vi "niVNA_SParamMeasure_Demo.vi"() -> ()   [LabVIEW 2013]
uses:
  <vilib>/Analysis/baseanly.llb/Mean (DBL).vi
  <instrlib>/niVNA/niVNA.llb/niVNA Load Calibration And Configuration Data From File.vi
  <instrlib>/niVNA/niVNA.llb/niVNA Fetch Sweep Measurement Complex (CDB).vi
  <vilib>/Analysis/baseanly.llb/Mean (CDB).vi
  <vilib>/Analysis/NI_AALBase.lvlib
panel:
  in  "Stop Button":bool
  out "P2":dbl[](graph)
  out "P1":dbl[](graph)
  out "CPD":dbl[](graph)
  out "error out":errorcluster
  in  "SavedCalPath":path=path "C:/Users/Eddie.Rickey/Documents/RCV_PXI/Calibration/#Cal - VNA_ 50MHz.chx"
  in  "resource name":refnum<k15>="5632_0"
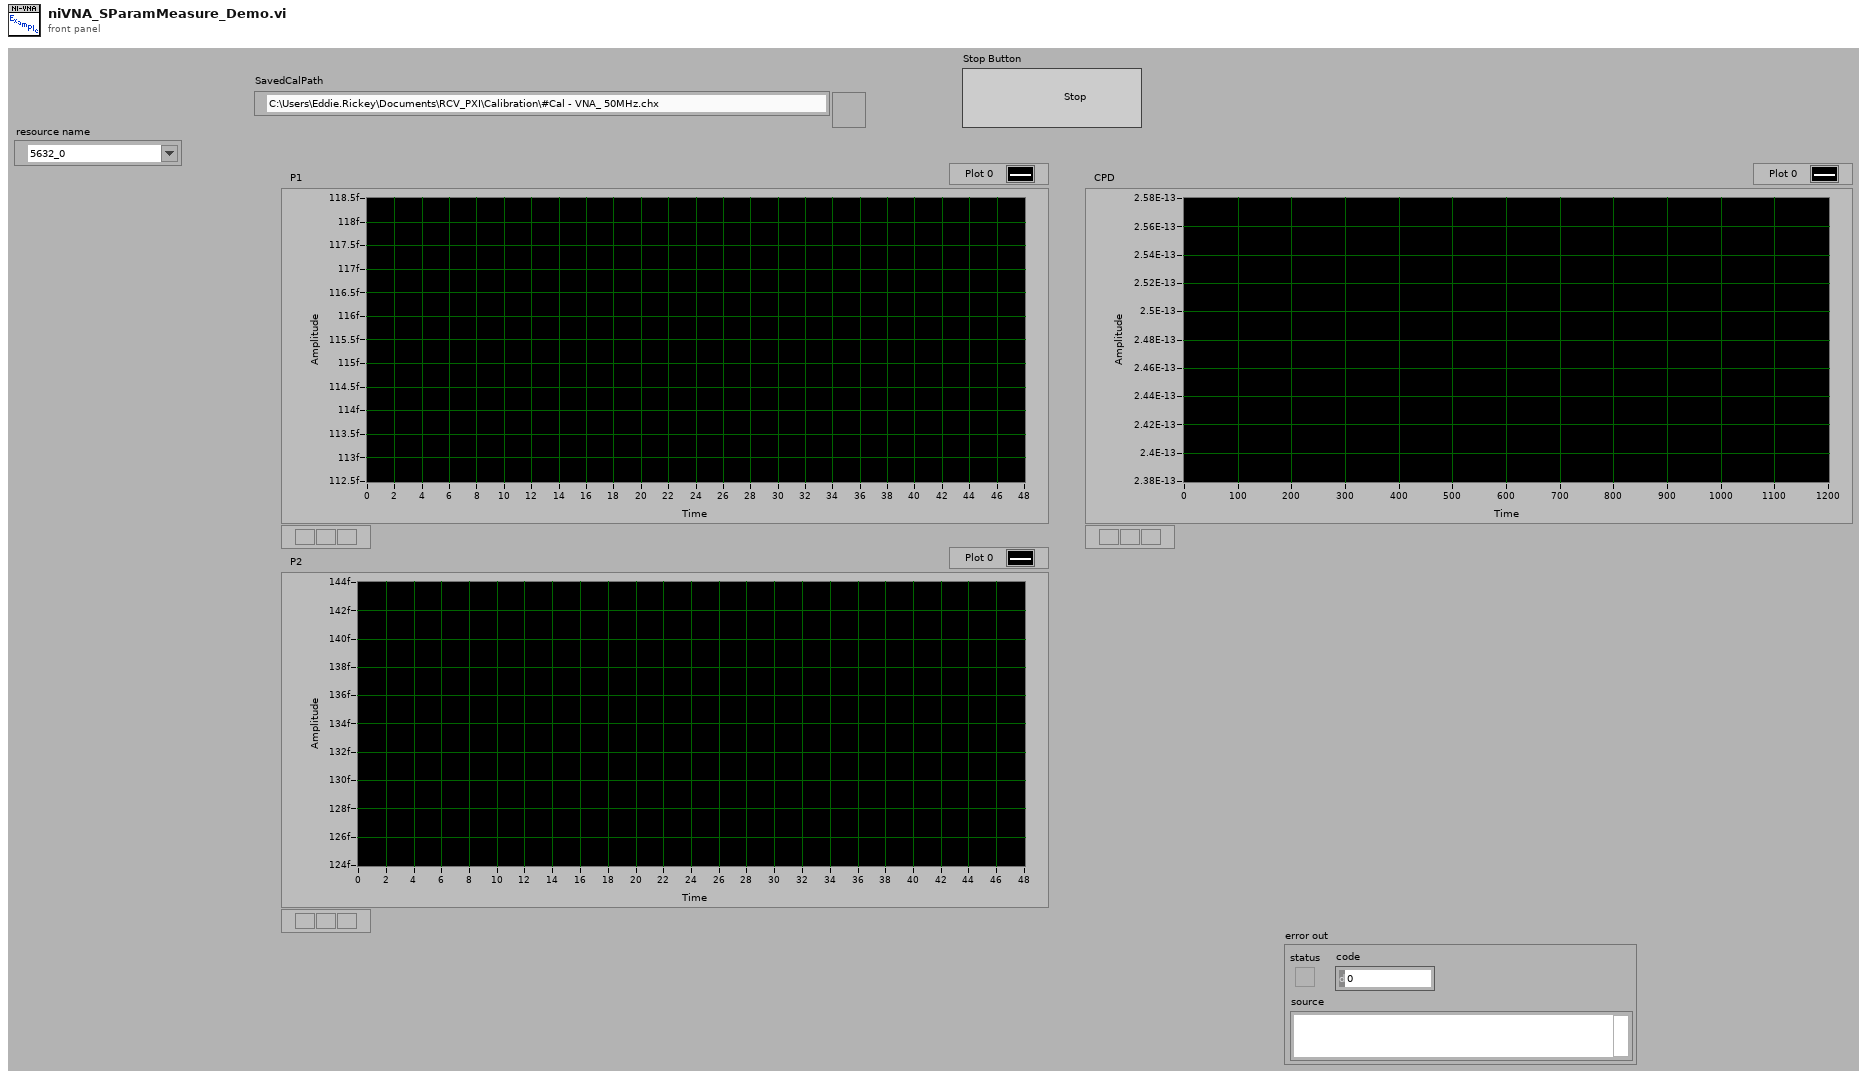
[diagram p1: front panel]
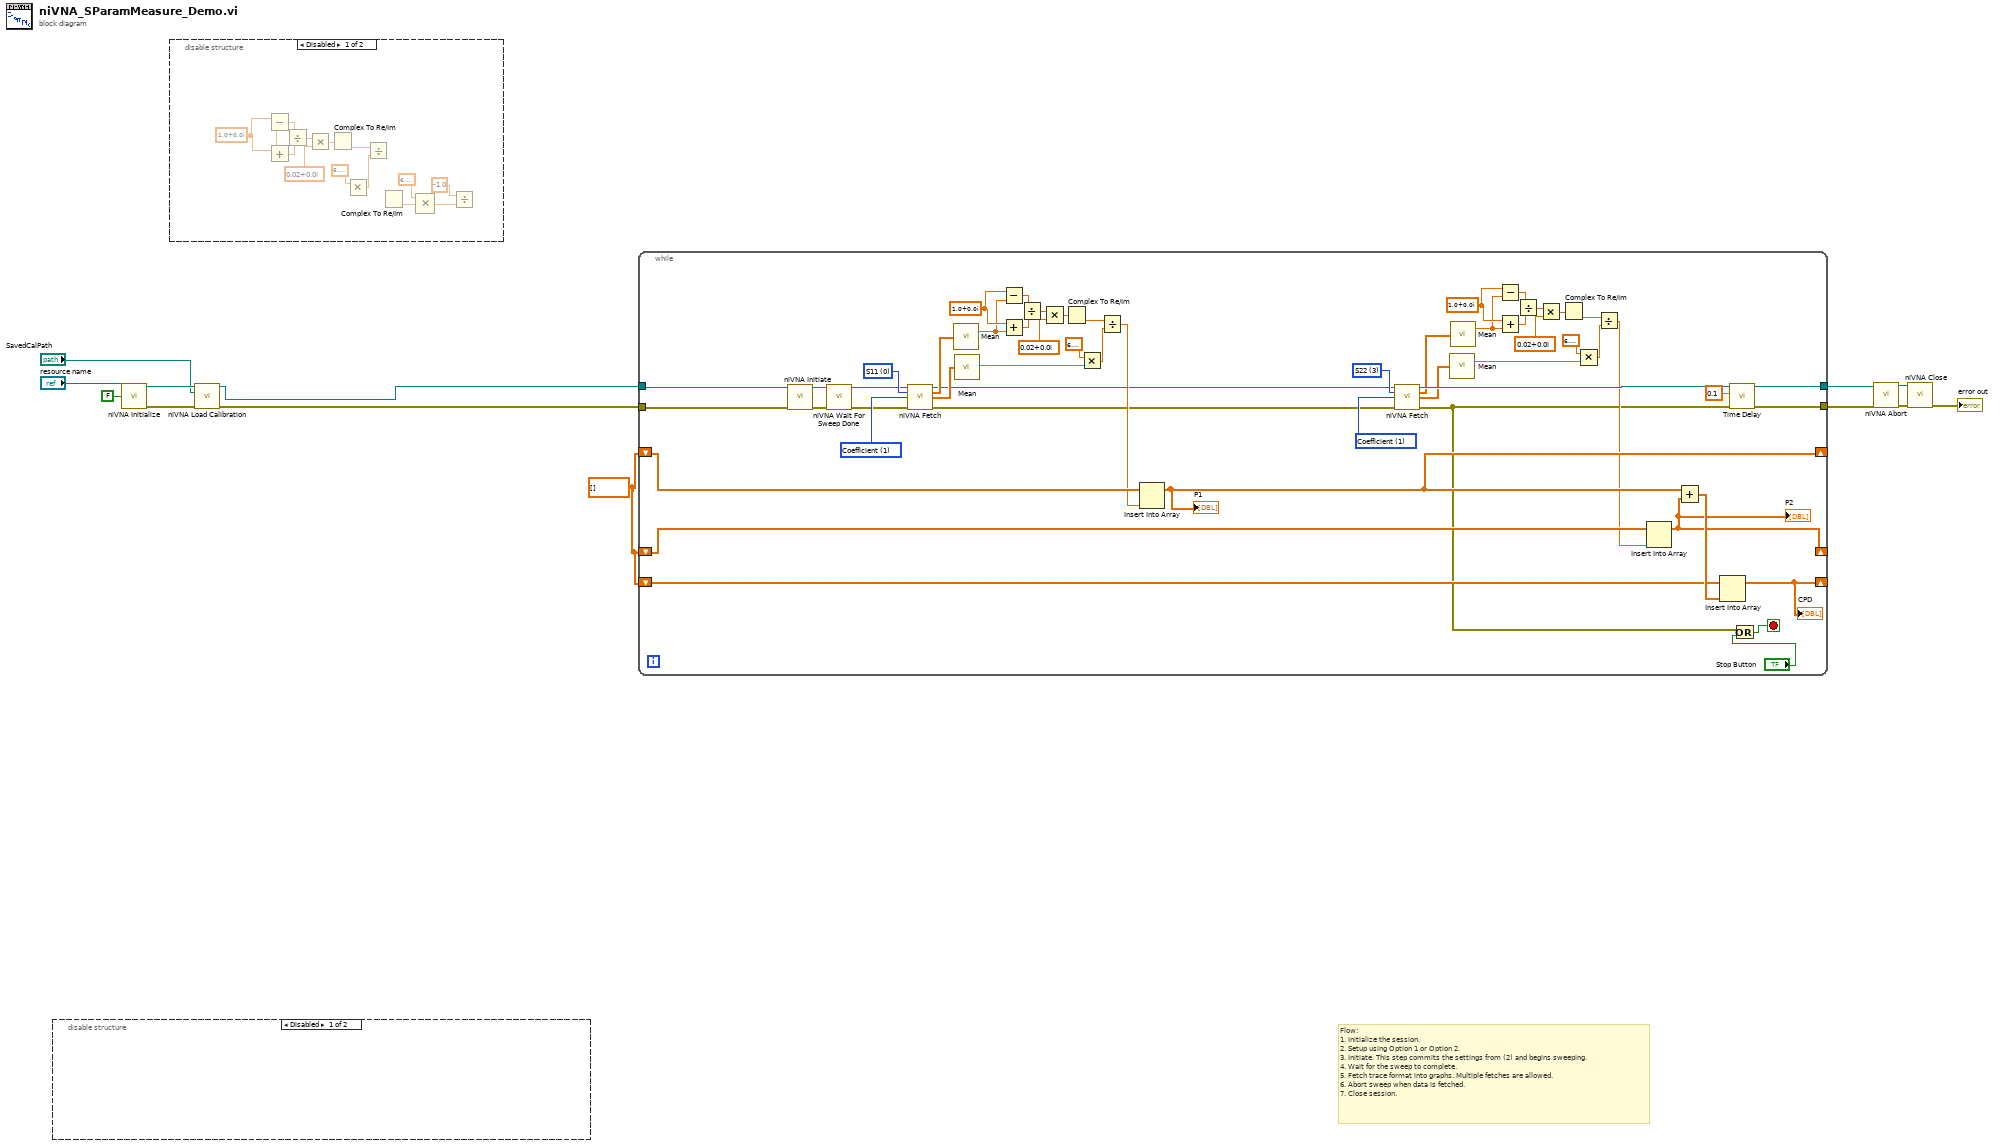
[diagram p0: block diagram]
diagram:
  w3 = dbl[] []
  # "Flow:\n1. Initialize the session.\n2. Setup using Option 1 or Option 2.\n3. Initiate. This step commits the settings from (2) and begins sweeping.\n4. Wait for the sweep to complete.\n5. Fetch trace format into graphs. Multiple fetches are allowed.\n6. Abort sweep when data is fetched.\n7. Close session."
  n1 = disable-structure shown="Disabled" {
    frame Disabled {
    }
    frame Enabled {
    }
  }
  n2 = call <instrlib>:"niVNA Initialize.vi"("resource name"="resource name", "reset"=FALSE) -> ("instrument handle"=w5:refnum<k15>, "error out"=w6:errorcluster)  [unwired: 12 in]
  n3 = disable-structure shown="Disabled" {
    frame Disabled {
      w28 = cdb 1.0+0.0i
      n4 = Subtract(x=w28) -> (y=w18:cdb, x-y=w27:cdb)
      n5 = Add(x=w28, y=w18) -> (x+y=w26:cdb)
      n6 = Divide(x=w27, y=w26) -> (x/y=w25:cdb)
      n7 = Multiply(x=w25, y=cdb 0.02+0.0i) -> (x*y=w23:cdb)
      n8 = Complex To Re/Im(x + iy=w23) -> (y=w21:dbl)  [unwired: 1 out]
      n9 = Multiply(x=6.283185307179586) -> (x*y=w20:dbl)  [unwired: 1 in]
      n10 = Divide(x=w21, y=w20) -> (x/y=w19:dbl)
      n11 = Complex To Re/Im() -> (y=w17:dbl)  [unwired: 1 in, 1 out]
      n12 = Compound Arithmetic op=MULTIPLY(6.283185307179586, w17) -> (w15:dbl)  [unwired: 1 in]
      n13 = Divide(x=-1.0, y=w15) -> ()  [unwired: 1 out]
    }
    frame Enabled {
    }
  }
  n14 = call-poly <instrlib>:"niVNA Load Calibration.vi"("instrument handle"=w5, "file path"="SavedCalPath", "error in"=w6) -> ("instrument handle out"=w1:refnum<k15>, "error out"=w2:errorcluster)  [unwired: 11 in]
  n15 = while {
    tunnel: [w81] -> w9
    tunnel: [w30] -> w8
    tunnel: w2 -> [w33]
    tunnel: w1 -> [w32]
    shift-right: [w71] -> _
    shift-left: w3 -> [w72]
    shift-right: [w66] -> _
    shift-left: w3 -> [w70]
    shift-right: [w68] -> _
    shift-left: w3 -> [w67]
    stop <- w80 stop-if-true
    w37 = 1 items=["Impedance", "Coefficient"] ("format")
    w53 = cdb 1.0+0.0i
    w65 = cdb 1.0+0.0i
    w36 = 3 items=["S11", "S21", "S12", "S22"] ("measurement")
    w78 = 1 items=["Impedance", "Coefficient"] ("format")
    w77 = 0 items=["S11", "S21", "S12", "S22"] ("measurement")
    n16 = call <instrlib>:"niVNA Initiate.vi"("instrument handle"=w32, "error in"=w33) -> ("instrument handle out"=w41:refnum<k15>, "error out"=w40:errorcluster)  [unwired: 12 in]
    n17 = call <instrlib>:"niVNA Wait For Sweep Done.vi"("instrument handle"=w41, "error in"=w40) -> ("instrument handle out"=w38:refnum<k15>, "error out"=w39:errorcluster)  [unwired: 12 in]
    n18 = call-poly <instrlib>:"niVNA Fetch.vi"("instrument handle"=w38, "measurement"=w77, "format"=w78, "error in"=w39) -> ("instrument handle out"=w34:refnum<k15>, "data"=w75:cdb[], "scale points"=w76:dbl[], "error out"=w35:errorcluster)  [unwired: 8 in]
    n19 = call-poly <vilib>:"Mean.vi"("X"=w75) -> ("mean"=w56:cdb)  [unwired: 1 out]
    n20 = call-poly <vilib>:"Mean.vi"("X"=w76) -> ("mean"=w55:dbl)  [unwired: 1 out]
    n21 = Subtract(x=w65, y=w56) -> (x-y=w64:cdb)
    n22 = Add(x=w65, y=w56) -> (x+y=w63:cdb)
    n23 = Divide(x=w64, y=w63) -> (x/y=w62:cdb)
    n24 = Multiply(x=w62, y=cdb 0.02+0.0i) -> (x*y=w60:cdb)
    n25 = Complex To Re/Im(x + iy=w60) -> (y=w58:dbl)  [unwired: 1 out]
    n26 = Multiply(x=6.283185307179586, y=w55) -> (x*y=w57:dbl)
    n27 = Divide(x=w58, y=w57) -> (x/y=w54:dbl)
    n28 = Insert Into Array(array=w72, new element=w54) -> (w71:dbl[])  [unwired: 1 in]
    "P1" <- w71
    n29 = call-poly <instrlib>:"niVNA Fetch.vi"("instrument handle"=w34, "measurement"=w36, "format"=w37, "error in"=w35) -> ("instrument handle out"=w81:refnum<k15>, "data"=w74:cdb[], "scale points"=w73:dbl[], "error out"=w31:errorcluster)  [unwired: 8 in]
    n30 = call-poly <vilib>:"Mean.vi"("X"=w73) -> ("mean"=w43:dbl)  [unwired: 1 out]
    n31 = call-poly <vilib>:"Mean.vi"("X"=w74) -> ("mean"=w44:cdb)  [unwired: 1 out]
    n32 = Subtract(x=w53, y=w44) -> (x-y=w52:cdb)
    n33 = Add(x=w53, y=w44) -> (x+y=w51:cdb)
    n34 = Divide(x=w52, y=w51) -> (x/y=w50:cdb)
    n35 = Multiply(x=w50, y=cdb 0.02+0.0i) -> (x*y=w48:cdb)
    n36 = Complex To Re/Im(x + iy=w48) -> (y=w46:dbl)  [unwired: 1 out]
    n37 = Multiply(x=6.283185307179586, y=w43) -> (x*y=w45:dbl)
    n38 = Divide(x=w46, y=w45) -> (x/y=w42:dbl)
    n39 = Insert Into Array(array=w70, new element=w42) -> (w66:dbl[])  [unwired: 1 in]
    "P2" <- w66
    n40 = Add(x=w71, y=w66) -> (x+y=w69:dbl[])
    n41 = Insert Into Array(array=w67, new element=w69) -> (w68:dbl[])  [unwired: 1 in]
    "CPD" <- w68
    n42 = call "Time Delay"("error in (no error)"=w31, "Delay Time (s)"=0.1) -> ("error out"=w30:errorcluster)  [unwired: 9 in]
    n43 = Or(x=w31, y="Stop Button") -> (x .or. y?=w80:bool)
  }
  n44 = call <instrlib>:"niVNA Abort.vi"("instrument handle"=w9, "error in"=w8) -> ("instrument handle out"=w11:refnum<k15>, "error out"=w10:errorcluster)  [unwired: 12 in]
  n45 = call <instrlib>:"niVNA Close.vi"("instrument handle"=w11, "error in"=w10) -> ("error out"=→"error out":errorcluster)  [unwired: 13 in]
